vi "FT Sensor.vi"() -> (0 "[Fx Fy Tz]":dbl[](array[numeric]))   [LabVIEW 2017]
uses:
  <vilib>/Utility/inputDevices.llb/joystickAcquire.vi
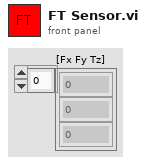
[diagram p1: front panel]
types:
  T1 = cluster{"X axis":i32, "Y axis":i32, "Z axis":i32, "X axis rotation":i32, "Y axis rotation":i32, "Z axis rotation":i32, "U axis":i32, "V axis":i32}
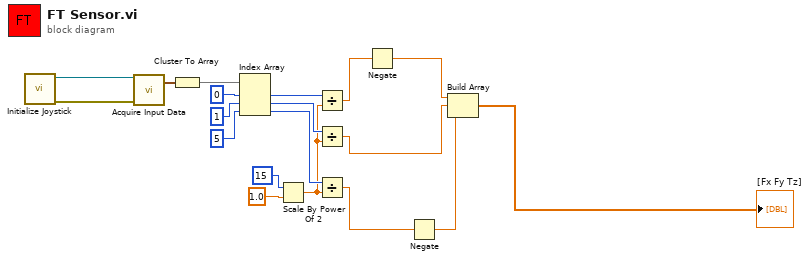
[diagram p0: block diagram]
diagram:
  n1 = call <vilib>:"Initialize Joystick.vi"() -> ("error out"=w6:errorcluster, "device ID"=w7:refnum<k1>)  [unwired: 10 in]
  n2 = call-poly <vilib>:"Acquire Input Data.vi"("device ID"=w7, "error in (no error)"=w6) -> ("axis info"=w18:T1)  [unwired: 13 in, 4 out]
  n3 = Cluster To Array(cluster=w18) -> (array=w14:i32[])
  n4 = Index Array(array=w14, index #1=0 ("index"), index #2=1 ("index"), index #3=5 ("index")) -> (element #1=w11:i32, element #2=w10:i32, element #3=w9:i32)
  n5 = Scale By Power Of 2(n=i16 15, x=1.0) -> (x*2^n=w8:dbl)
  n6 = Divide(x=w11, y=w8) -> (x/y=w5:dbl)
  n7 = Divide(x=w10, y=w8) -> (x/y=w3:dbl)
  n8 = Divide(x=w9, y=w8) -> (x/y=w2:dbl)
  n9 = Negate(x=w5) -> (-x=w4:dbl)
  n10 = Negate(x=w2) -> (-x=w1:dbl)
  n11 = Build Array(w4, w3, w1) -> (→"[Fx Fy Tz]":dbl[])
